vi "SPIM Controller 2016.vi"() -> ()   [LabVIEW 2016]
uses:
  controls/Microscope Settings.ctl
  controls/CameraControlTypeDef.ctl
  controls/ModeEnum.ctl
panel:
  in  "File Path Control":path
  in  "Add Settings":bool
  out "error IO":errorcluster
  out "Duration":string
  in  "Scans":dbl=1.0 min=0.0 max=10.0 step=0.05
  in  "Scan":bool
  in  "Scan Cont":bool
  in  "Multicolumn Listbox":i32(listbox)
  in  "stop":bool
  in  "Load Settings":bool
  in  "Save Settings":bool
  in  "Record":bool
  in  "Signals Debugger":bool
  in  "Stage Controller":bool
  in  "Microscope Settings":T1={"Mode"=enum."XY", "Slit"={"Scanning Mode"=12.0, "Slit Width /%"=5.0}, "Colour"=[{"Laser"=enum."561", "Filter"=4}], "Exposure/ms"=40.0, "Piezo Position /um"=0.0, "ROI"={"X"={"Start /px"=0.0, "Step /px"=1.0, "Range /px"=2048.0}, "Y"={"Start /px"=0.0, "Step /px"=1.0, "Range /px"=2048.0}, "Z "={"Start /um"=0.0, "Step/um"=1.0, "Range /um"=100.0}, "T "={"Start /s"=0.0, "Step /s"=1.0, "Range /s"=100.0}}, "Samples per millisecond"=100.0, "Relax/ms"=10.0, "Readout Direction"=2.0, "Trigger Source"=2.0, "Camera Delay /ms"=11.0, "Under Scan /ms"=5.0, "Calibration Coordinates"={"Top Left"=[-4.418670520231216, -0.1592138728323702, 10.0], "Top Right"=[-9.501965317919073, -0.1592138728323702, 10.0], "Bottom Left"=[-4.4508670520231215, 0.0, 0.0], "Bottom Right"=[-9.53757225433526, 0.0, 0.0], "Waveforms"={"Analogue Out"=[], "Digital Out"=[]}}} {"Under Scan /ms" min=0.0 max=10.0 step=0.05; "ROI"."T"."Range /s" min=0.0 max=10.0 step=0.05 format="%<%H:%M:%S>t"; "ROI"."T"."Step /s" min=0.0 max=10.0 step=0.05 format="%<%M:%S%2u>t"; "ROI"."T"."Start /s" min=0.0 max=10.0 step=0.05 format="%<%M:%S%2u>t"; "ROI"."X"."Range /px" min=0.0 max=10.0 step=0.05; "ROI"."X"."Step /px" min=0.0 max=10.0 step=0.05; "ROI"."X"."Start /px" min=0.0 max=10.0 step=0.05; "ROI"."Y"."Range /px" min=0.0 max=10.0 step=0.05; "ROI"."Y"."Step /px" min=0.0 max=10.0 step=0.05; "ROI"."Y"."Start /px" min=0.0 max=10.0 step=0.05; "ROI"."Z"."Range /um" min=0.0 max=10.0 step=0.05; "ROI"."Z"."Step/um" min=0.0001 max=10.0 step=0.05; "ROI"."Z"."Start /um" min=0.0 max=10.0 step=0.05; "Colour"."Filter" items=["Empty"=1, ""=2, ""=3, "561"=4, ""=5, "488"=6]; "Camera Delay /ms" min=0.0 max=10.0 step=0.05; "Trigger Source" items=["Internal"=1.0, "External"=2.0]; "Readout Direction" items=["Forward"=1.0, "Backward"=2.0]; "Slit"."Scanning Mode" items=["Full Frame"=1.0, "Slit Scanning"=12.0]; "Piezo Position /um" min=0.0 max=10.0 step=0.05}
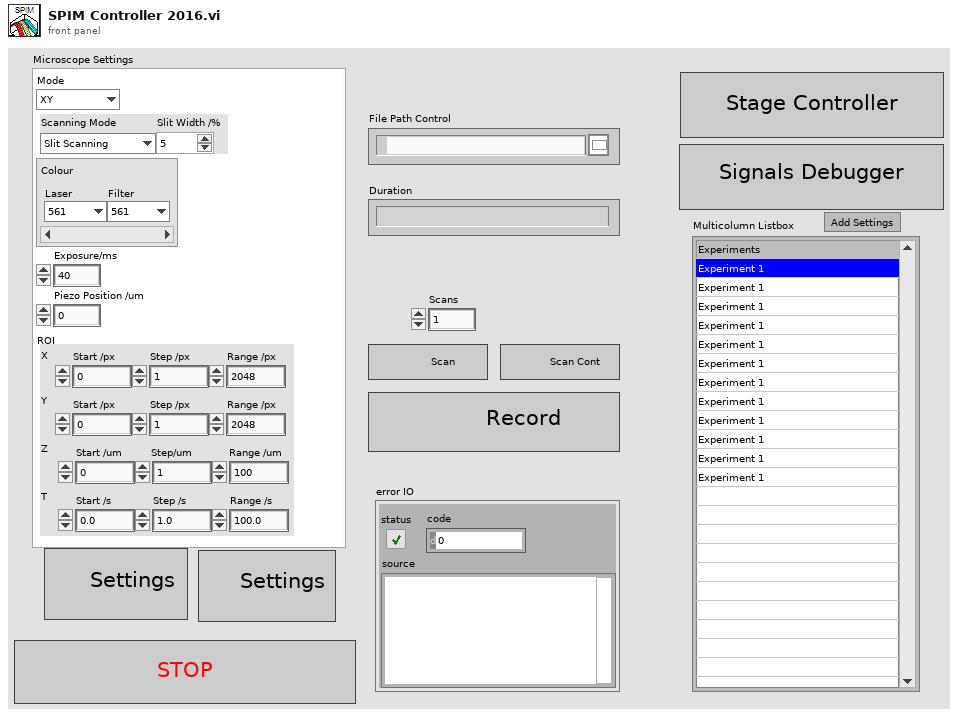
[diagram p1: front panel]
types:
  T1 = typedef "Microscope Settings.ctl" = cluster{"Mode":enum16{"Brightfield", "X", "XY", "XYZ", "XYZT", "XYZC", "Tweezers", "Virus"}, "Slit":cluster{"Scanning Mode":dbl, "Slit Width /%":dbl}, "Colour":cluster{"Laser":enum16{"Brightfield", "445", "488", "561", "647"}, "Filter":u16}[], "Exposure/ms":dbl, "Piezo Position /um":dbl, "ROI":cluster{"X":cluster{"Start /px":dbl, "Step /px":dbl, "Range /px":dbl}, "Y":cluster{"Start /px":dbl, "Step /px":dbl, "Range /px":dbl}, "Z ":cluster{"Start /um":dbl, "Step/um":dbl, "Range /um":dbl}, "T ":cluster{"Start /s":dbl, "Step /s":dbl, "Range /s":dbl}}, "Samples per millisecond":dbl, "Relax/ms":dbl, "Readout Direction":dbl, "Trigger Source":dbl, "Camera Delay /ms":dbl, "Under Scan /ms":dbl, "Calibration Coordinates":cluster{"Top Left":dbl[], "Top Right":dbl[], "Bottom Left":dbl[], "Bottom Right":dbl[], "Waveforms":cluster{"Analogue Out":waveform(dbl)[], "Digital Out":digitalwaveform[]}}}
  T2 = typedef "ModeEnum.ctl" = enum16{"Idle", "Init", "generateWaves", "runWaves", "runWavesCont", "endWavesCont", "stop"}
  T3 = typedef "CameraControlTypeDef.ctl" = enum16{"Idle", "Init", "Close", "IntervalLineInt", "Ram Record", "HardDisk Record", "Disengage Update", "Update", "ROI", "Binning", "Scan Mode", "Trigger Mode", "Readout Mode", "Readout Direction", "Preview", "ROIWindow", "Trigger Source"}
  T4 = enum32{"Invalid", "Standard", "Closed", "Hidden", "Minimized", "Maximized"}
  T5 = enum16{"open", "replace", "create", "open or create", "replace or create", "replace or create with confirmation"}
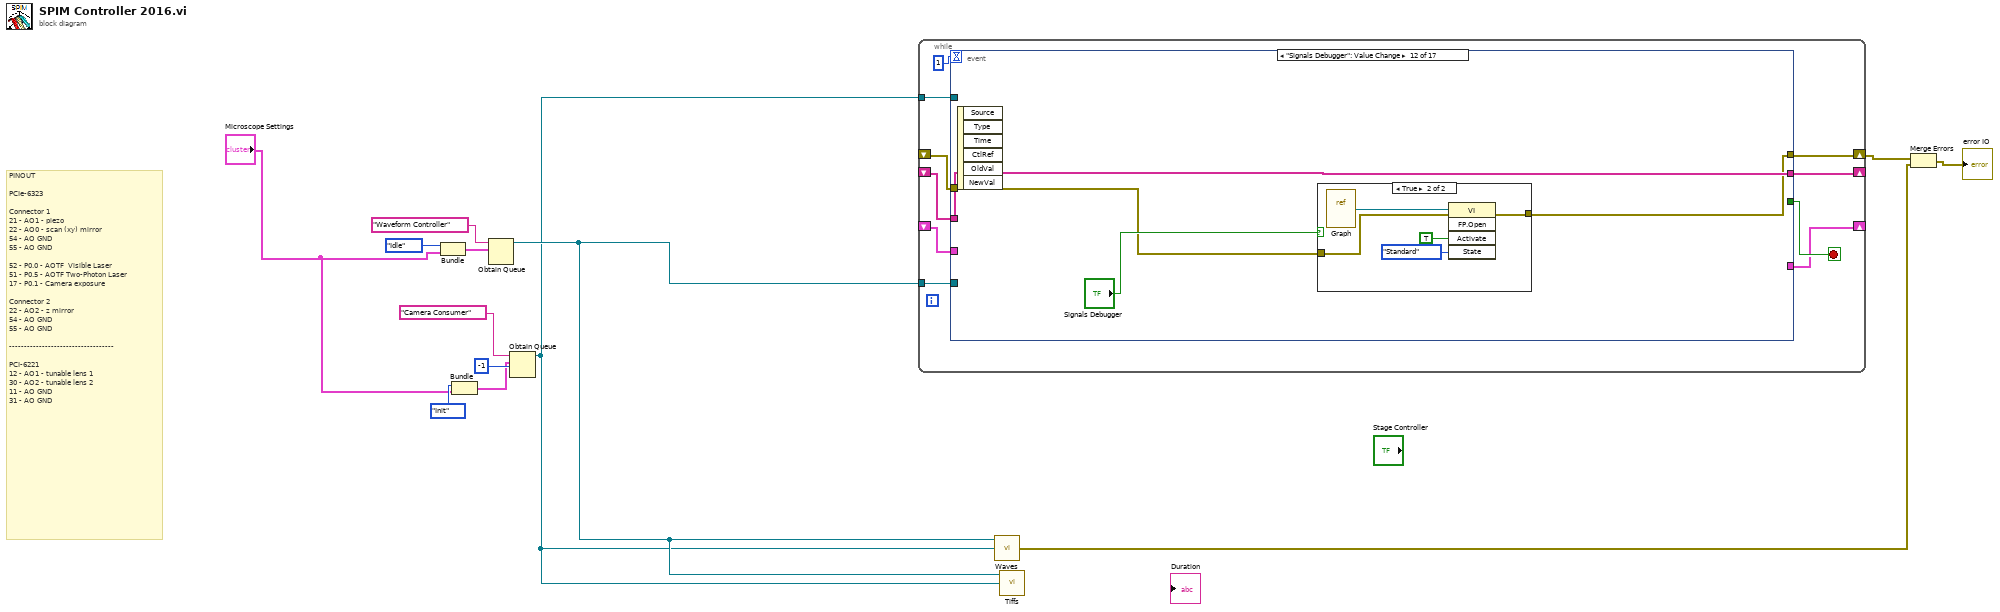
[diagram p0: block diagram]
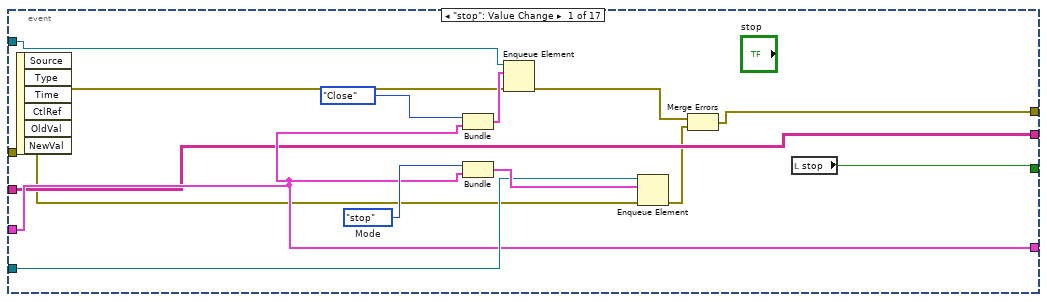
[diagram p2: hidden frame]
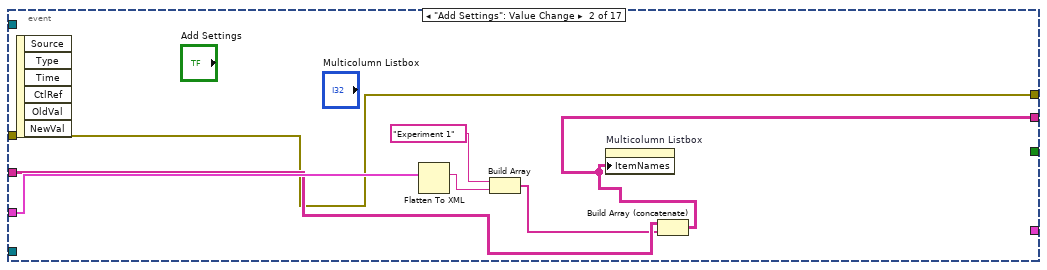
[diagram p3: hidden frame]
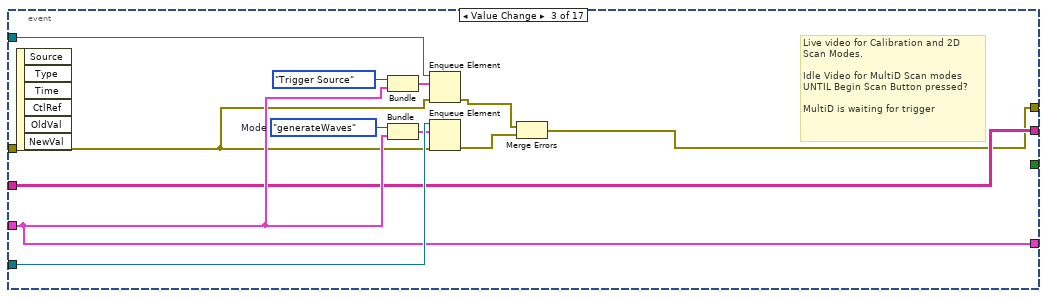
[diagram p4: hidden frame]
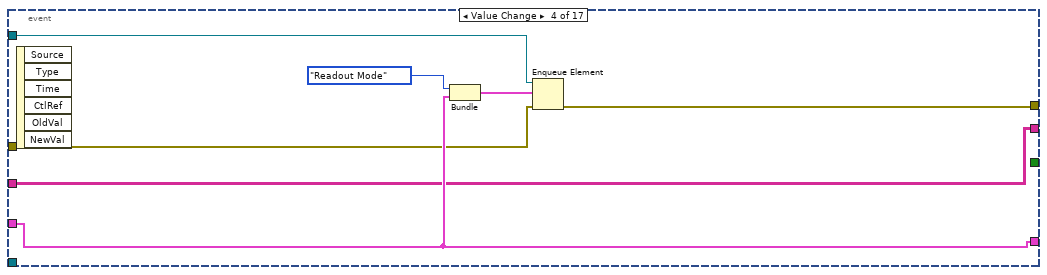
[diagram p5: hidden frame]
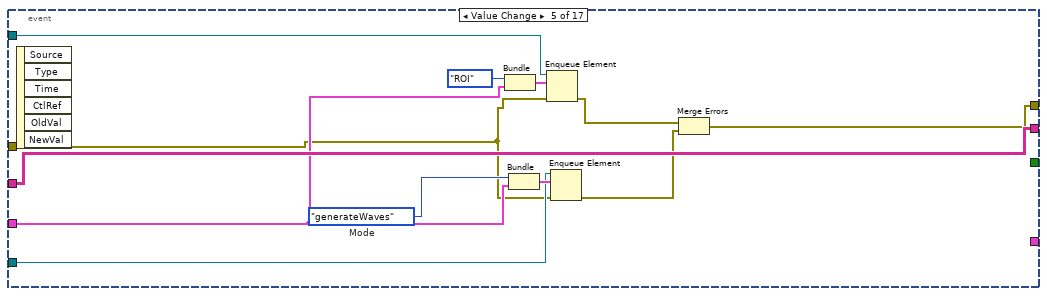
[diagram p6: hidden frame]
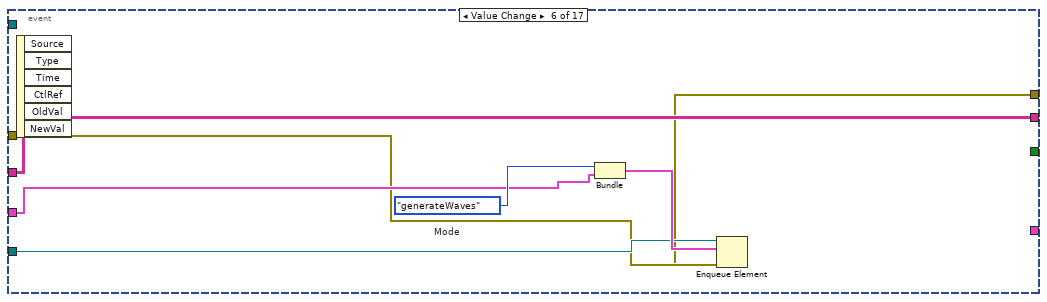
[diagram p7: hidden frame]
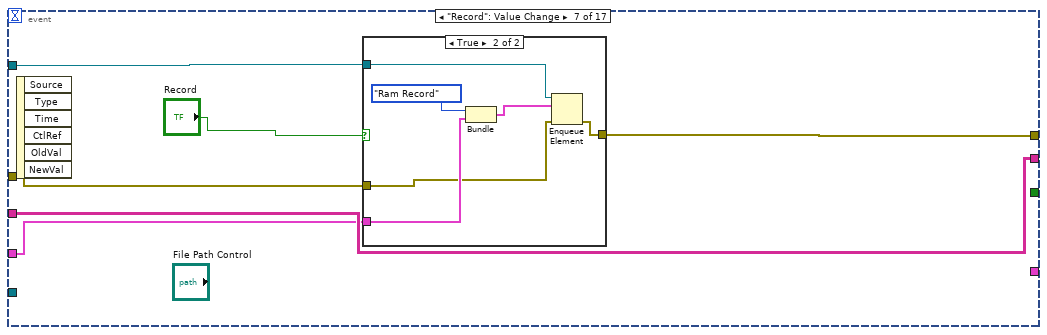
[diagram p8: hidden frame]
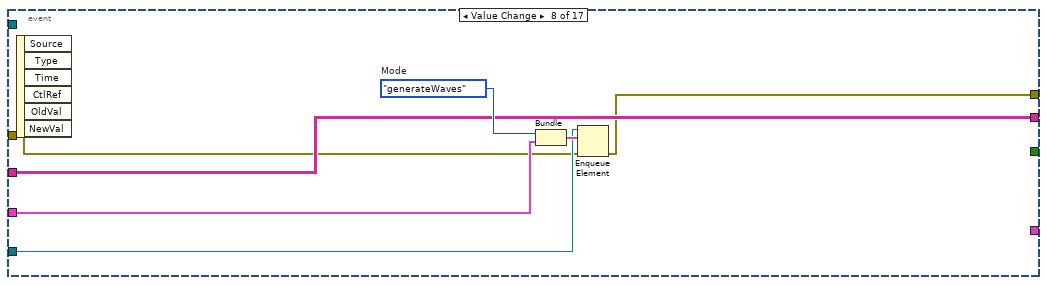
[diagram p10: hidden frame]
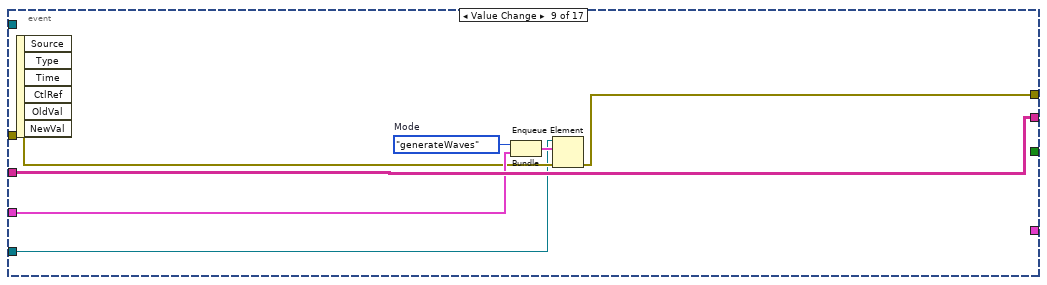
[diagram p11: hidden frame]
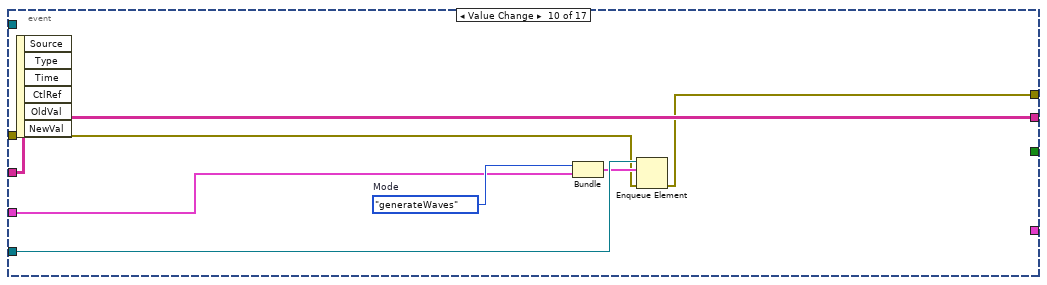
[diagram p12: hidden frame]
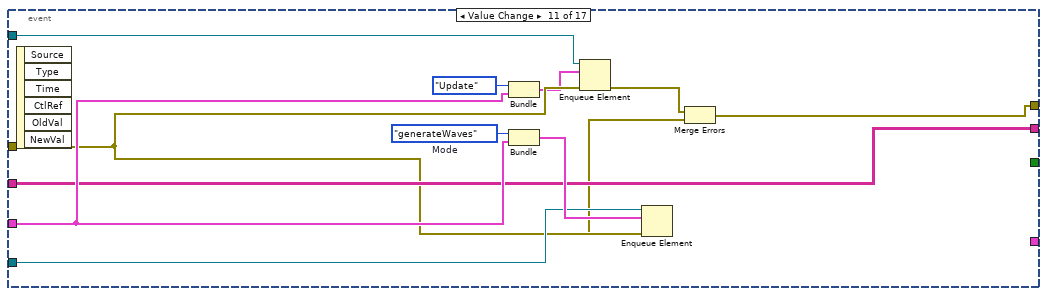
[diagram p13: hidden frame]
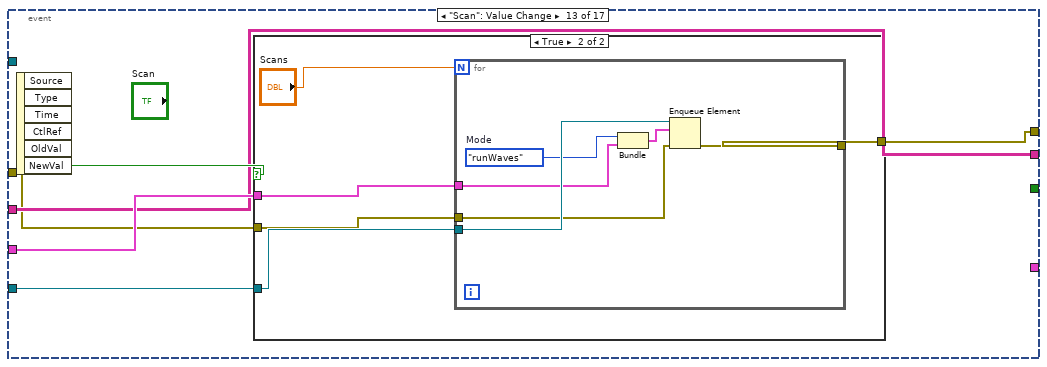
[diagram p15: hidden frame]
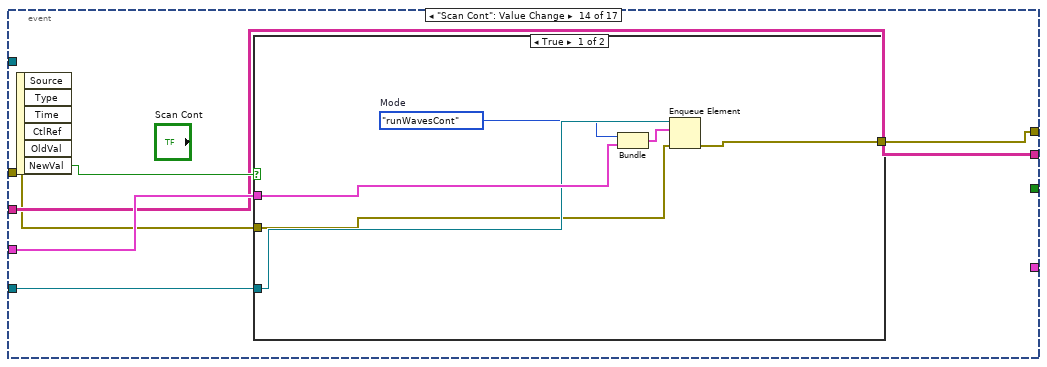
[diagram p17: hidden frame]
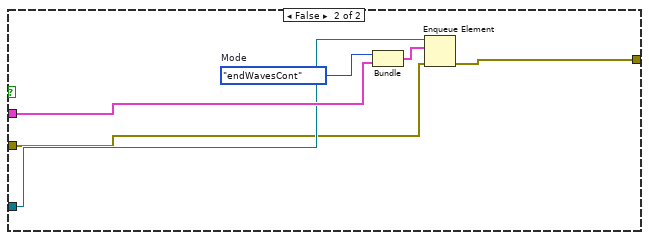
[diagram p18: hidden frame]
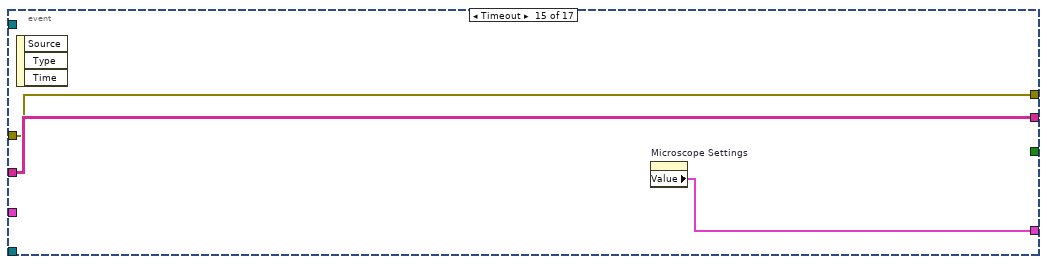
[diagram p19: hidden frame]
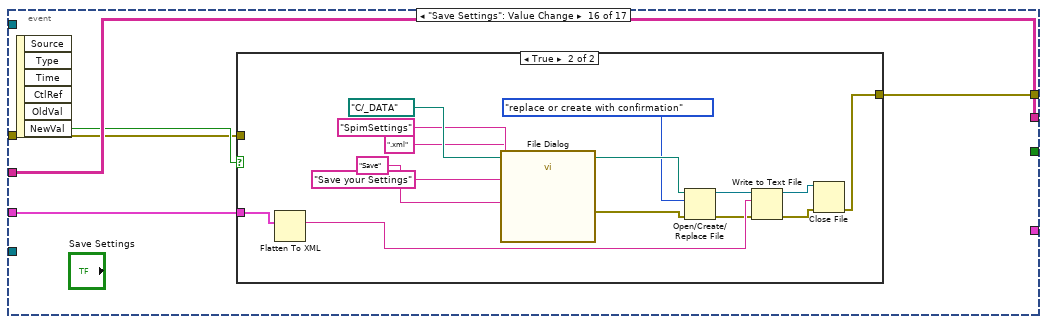
[diagram p20: hidden frame]
diagram:
  # "PINOUT\n\nPCIe-6323\n\nConnector 1\n21 - AO1 - piezo\n22 - AO0 - scan (xy) mirror\n54 - AO GND\n55 - AO GND\n\n52 - P0.0 - AOTF  Visible Laser\n51 - P0.5 - AOTF Two-Photon Laser\n17 - P0.1 - Camera exposure\n\nConnector 2\n22 - AO2 - z mirror\n54 - AO GND\n55 - AO GND\n\n-----------------------------------\n\nPCI-6221\n12 - AO1 - tunable lens 1\n30 - AO2 - tunable lens 2\n11 - AO GND\n31 - AO GND"
  n1 = Bundle("Mode"=ModeEnum."Idle", "Microscope Settings"="Microscope Settings") -> (w8:cluster{"Mode":T2, "Microscope Settings":T1})  [unwired: 1 in]
  n2 = Bundle("Enum"=CameraControlTypeDef."Init", "Microscope Settings"="Microscope Settings") -> (w10:cluster{"Enum":T3, "Microscope Settings":T1})  [unwired: 1 in]
  n3 = Obtain Queue(name (unnamed)="Waveform Controller", element data type=w8) -> (queue out=w6:refnum<queue>)  [unwired: 3 in, 2 out]
  n4 = Obtain Queue(max queue size (-1, unlimited)=-1, name (unnamed)="Camera Consumer", element data type=w10) -> (queue out=w5:refnum<queue>)  [unwired: 2 in, 2 out]
  n5 = while {
    tunnel: w5 -> [w22]
    shift-right: [w21] -> _
    shift-left: _ -> [w20]
    tunnel: w6 -> [w18]
    shift-right: [w17] -> _
    shift-left: _ -> [w16]
    shift-right: [w15] -> w3
    shift-left: _ -> [w14]
    stop <- w23 stop-if-true
    n6 = event shown="[11] \"Signals Debugger\": Value Change" {
      selector: _ -> [_ _ _ _ _ _ _ _ _ _ _ _ _ _ _ _ _]
      dyn-events: _ -> [_ _ _ _ _ _ _ _ _ _ _ _ _ _ _ _ _]
      timeout: 1 -> [_ _ _ _ _ _ _ _ _ _ _ _ _ _ _ _ _]
      tunnel: [w36 _ _ _ _ _ _ _ _ _ _ _ _ _ _ _ _] -> w23
      tunnel: w22 -> [w24 _ w44 w56 w63 _ w86 _ _ _ w116 _ _ _ _ _ _]
      tunnel: [w30 _ w50 w61 _ _ _ _ _ _ _ _ _ _ w176 _ w199] -> w21
      tunnel: w20 -> [w30 w43 w50 w61 w69 w77 w85 w99 w106 w112 w124 _ w143 w161 _ w180 w200]
      tunnel: w18 -> [w31 _ w55 _ w70 w78 _ w98 w102 w113 w123 _ w142 w160 _ _ _]
      tunnel: [w29 w38 w49 w59 w72 w81 w87 w97 w108 w115 w122 w131 w140 w158 w175 w181 w201] -> w17
      tunnel: w16 -> [w29 w40 w49 w59 w72 w81 w87 w97 w108 w115 w122 w131 w140 w158 w175 w181 w201]
      tunnel: [w25 w37 w45 w57 w64 w75 w83 w95 w104 w110 w118 w129 w139 w157 w174 w179 _] -> w15
      tunnel: w14 -> [w28 w37 w48 w58 w67 w76 w84 w96 w105 w109 w121 w128 w138 w156 w174 w177 _]
      event "stop": Value Change {
        w34 = ModeEnum."stop"  # Mode
        n7 = event-data() -> ()  [unwired: 1 in, 6 out]
        n8 = Bundle("Enum"=CameraControlTypeDef."Close", "Value"=w30) -> (w32:cluster{"Enum":T3, "Value":T1})  [unwired: 1 in]
        n9 = Bundle("Mode"=w34, "Value"=w30) -> (w33:cluster{"Mode":T2, "Value":T1})  [unwired: 1 in]
        n10 = Enqueue Element(queue=w24, element=w32, error in (no error)=w28) -> (error out=w26:errorcluster)  [unwired: 1 in, 2 out]
        n11 = Enqueue Element(queue=w31, element=w33, error in (no error)=w28) -> (error out=w27:errorcluster)  [unwired: 1 in, 2 out]
        n12 = Merge Errors(w26, w27) -> (w25:errorcluster)
        n13 = local read "stop"() -> (w36:bool)
      }
      event "Add Settings": Value Change {
        n14 = event-data() -> ()  [unwired: 1 in, 6 out]
        n15 = Flatten To XML(anything=w43) -> (xml string=w42:string)
        n16 = Build Array("Experiment 1" ("element"), w42) -> (w39:string[])
        n17 = Build Array (concatenate)(w40, w39) -> (w38:string[][])
        n18 = property on="Multicolumn Listbox" class="MCListbox (strict)"("ItemNames"=w38) -> ()  [unwired: 2 in, 2 out]
      }
      event Value Change {
        w53 = ModeEnum."generateWaves"  # Mode
        # "Live video for Calibration and 2D\nScan Modes.\n\nIdle Video for MultiD Scan modes\nUNTIL Begin Scan Button pressed?\n\nMultiD is waiting for trigger"
        n19 = event-data() -> ()  [unwired: 1 in, 6 out]
        n20 = Bundle("Enum"=CameraControlTypeDef."Trigger Source", "Value"=w50) -> (w51:cluster{"Enum":T3, "Value":T1})  [unwired: 1 in]
        n21 = Bundle("Mode"=w53, "Value"=w50) -> (w52:cluster{"Mode":T2, "Value":T1})  [unwired: 1 in]
        n22 = Enqueue Element(queue=w44, element=w51, error in (no error)=w48) -> (error out=w46:errorcluster)  [unwired: 1 in, 2 out]
        n23 = Enqueue Element(queue=w55, element=w52, error in (no error)=w48) -> (error out=w47:errorcluster)  [unwired: 1 in, 2 out]
        n24 = Merge Errors(w46, w47) -> (w45:errorcluster)
      }
      event Value Change {
        n25 = event-data() -> ()  [unwired: 1 in, 6 out]
        n26 = Bundle("Enum"=CameraControlTypeDef."Readout Mode", "Value"=w61) -> (w60:cluster{"Enum":T3, "Value":T1})  [unwired: 1 in]
        n27 = Enqueue Element(queue=w56, element=w60, error in (no error)=w58) -> (error out=w57:errorcluster)  [unwired: 1 in, 2 out]
      }
      event Value Change {
        w68 = ModeEnum."generateWaves"  # Mode
        n28 = event-data() -> ()  [unwired: 1 in, 6 out]
        n29 = Bundle("Enum"=CameraControlTypeDef."ROI", "Value"=w69) -> (w73:cluster{"Enum":T3, "Value":T1})  [unwired: 1 in]
        n30 = Bundle("Mode"=w68, "Value"=w69) -> (w71:cluster{"Mode":T2, "Value":T1})  [unwired: 1 in]
        n31 = Enqueue Element(queue=w63, element=w73, error in (no error)=w67) -> (error out=w65:errorcluster)  [unwired: 1 in, 2 out]
        n32 = Enqueue Element(queue=w70, element=w71, error in (no error)=w67) -> (error out=w66:errorcluster)  [unwired: 1 in, 2 out]
        n33 = Merge Errors(w65, w66) -> (w64:errorcluster)
      }
      event Value Change {
        w79 = ModeEnum."generateWaves"  # Mode
        n34 = event-data() -> ()  [unwired: 1 in, 6 out]
        n35 = Bundle("Mode"=w79, "Value"=w77) -> (w80:cluster{"Mode":T2, "Value":T1})  [unwired: 1 in]
        n36 = Enqueue Element(queue=w78, element=w80, error in (no error)=w76) -> (error out=w75:errorcluster)  [unwired: 1 in, 2 out]
      }
      event "Record": Value Change {
        n37 = event-data() -> ()  [unwired: 1 in, 6 out]
        n38 = case shown="True" "Record" {
          tunnel: w86 -> [_ w89]
          tunnel: w85 -> [_ w93]
          tunnel: w84 -> [w88 w91]
          tunnel: [w88 w90] -> w83
          frame False {
          }
          frame True {
            n39 = Bundle("Enum"=CameraControlTypeDef."Ram Record", "Value"=w93) -> (w92:cluster{"Enum":T3, "Value":T1})  [unwired: 1 in]
            n40 = Enqueue Element(queue=w89, element=w92, error in (no error)=w91) -> (error out=w90:errorcluster)  [unwired: 1 in, 2 out]
          }
        }
      }
      event Value Change {
        w101 = ModeEnum."generateWaves"  # Mode
        n41 = event-data() -> ()  [unwired: 1 in, 6 out]
        n42 = Bundle("Mode"=w101, "Value"=w99) -> (w100:cluster{"Mode":T2, "Value":T1})  [unwired: 1 in]
        n43 = Enqueue Element(queue=w98, element=w100, error in (no error)=w96) -> (error out=w95:errorcluster)  [unwired: 1 in, 2 out]
      }
      event Value Change {
        w107 = ModeEnum."generateWaves"  # Mode
        n44 = event-data() -> ()  [unwired: 1 in, 6 out]
        n45 = Bundle("Mode"=w107, "Value"=w106) -> (w103:cluster{"Mode":T2, "Value":T1})  [unwired: 1 in]
        n46 = Enqueue Element(queue=w102, element=w103, error in (no error)=w105) -> (error out=w104:errorcluster)  [unwired: 1 in, 2 out]
      }
      event Value Change {
        w114 = ModeEnum."generateWaves"  # Mode
        n47 = event-data() -> ()  [unwired: 1 in, 6 out]
        n48 = Bundle("Mode"=w114, "Value"=w112) -> (w111:cluster{"Mode":T2, "Value":T1})  [unwired: 1 in]
        n49 = Enqueue Element(queue=w113, element=w111, error in (no error)=w109) -> (error out=w110:errorcluster)  [unwired: 1 in, 2 out]
      }
      event Value Change {
        w126 = ModeEnum."generateWaves"  # Mode
        n50 = event-data() -> ()  [unwired: 1 in, 6 out]
        n51 = Bundle("Enum"=CameraControlTypeDef."Update", "Value"=w124) -> (w117:cluster{"Enum":T3, "Value":T1})  [unwired: 1 in]
        n52 = Bundle("Mode"=w126, "Value"=w124) -> (w125:cluster{"Mode":T2, "Value":T1})  [unwired: 1 in]
        n53 = Enqueue Element(queue=w116, element=w117, error in (no error)=w121) -> (error out=w120:errorcluster)  [unwired: 1 in, 2 out]
        n54 = Enqueue Element(queue=w123, element=w125, error in (no error)=w121) -> (error out=w119:errorcluster)  [unwired: 1 in, 2 out]
        n55 = Merge Errors(w120, w119) -> (w118:errorcluster)
      }
      event "Signals Debugger": Value Change {
        n56 = event-data() -> ()  [unwired: 1 in, 6 out]
        n57 = case shown="True" "Signals Debugger" {
          tunnel: [w132 w134] -> w129
          tunnel: w128 -> [w132 w133]
          frame False {
          }
          frame True {
            n58 = vi-ref "Graph.vi"() -> (w135:refnum<vi>)
            n59 = invoke class="VI" method="FP.Open"(reference=w135, error in=w133, "Activate"=TRUE ("Front Panel Window:Open"), "State"=T4."Standard") -> (error out=w134:errorcluster)  [unwired: 1 in, 4 out]
          }
        }
      }
      event "Scan": Value Change {
        n60 = event-data() -> ("NewVal"=w141:bool)  [unwired: 1 in, 5 out]
        n61 = case shown="True" w141 {
          tunnel: w143 -> [_ w149]
          tunnel: w142 -> [_ w148]
          tunnel: [w144 w147] -> w139
          tunnel: w138 -> [w144 w146]
          frame False {
          }
          frame True {
            n62 = for {
              N: "Scans" -> [_]
              tunnel: w149 -> [w152]
              tunnel: w148 -> [w155]
              tunnel: [w151] -> w147
              tunnel: w146 -> [w150]
              w154 = ModeEnum."runWaves"  # Mode
              n63 = Bundle("Mode"=w154, "Value"=w152) -> (w153:cluster{"Mode":T2, "Value":T1})  [unwired: 1 in]
              n64 = Enqueue Element(queue=w155, element=w153, error in (no error)=w150) -> (error out=w151:errorcluster)  [unwired: 1 in, 2 out]
            }
          }
        }
      }
      event "Scan Cont": Value Change {
        n65 = event-data() -> ("NewVal"=w159:bool)  [unwired: 1 in, 5 out]
        n66 = case shown="True" w159 {
          tunnel: w161 -> [w167 w173]
          tunnel: w160 -> [w166 w172]
          tunnel: [w165 w171] -> w157
          tunnel: w156 -> [w164 w170]
          frame True {
            w163 = ModeEnum."runWavesCont"  # Mode
            n67 = Bundle("Mode"=w163, "Value"=w167) -> (w162:cluster{"Mode":T2, "Value":T1})  [unwired: 1 in]
            n68 = Enqueue Element(queue=w166, element=w162, error in (no error)=w164) -> (error out=w165:errorcluster)  [unwired: 1 in, 2 out]
          }
          frame False {
            w169 = ModeEnum."endWavesCont"  # Mode
            n69 = Bundle("Mode"=w169, "Value"=w173) -> (w168:cluster{"Mode":T2, "Value":T1})  [unwired: 1 in]
            n70 = Enqueue Element(queue=w172, element=w168, error in (no error)=w170) -> (error out=w171:errorcluster)  [unwired: 1 in, 2 out]
          }
        }
      }
      event Timeout {
        n71 = event-data() -> ()  [unwired: 1 in, 3 out]
        n72 = property on="Microscope Settings" class="Clust (strict)"() -> ("Value"=w176:T1)  [unwired: 2 in, 2 out]
      }
      event "Save Settings": Value Change {
        n73 = event-data() -> ("NewVal"=w178:bool)  [unwired: 1 in, 5 out]
        n74 = case shown="True" w178 {
          tunnel: w180 -> [_ w197]
          tunnel: [w182 w185] -> w179
          tunnel: w177 -> [w182 _]
          frame False {
          }
          frame True {
            n75 = Flatten To XML(anything=w197) -> (xml string=w190:string)
            n76 = call "File Dialog"("start path"=path "C:/_DATA", "prompt"="Save your Settings", "button label"="Save", "default name"="SpimSettings", "pattern (all files)"=".xml") -> ("selected path"=w191:path, "error out"=w184:errorcluster)  [unwired: 7 in, 2 out]
            n77 = Open/Create/Replace File(file path (use dialog)=w191, error in=w184, operation (0:open)=T5."replace or create with confirmation") -> (refnum out=w189:refnum<file>, error out=w186:errorcluster)  [unwired: 3 in, 1 out]
            n78 = Write to Text File(file (use dialog)=w189, text=w190, error in=w186) -> (refnum out=w188:refnum<file>, error out=w187:errorcluster)  [unwired: 1 in, 1 out]
            n79 = Close File(refnum=w188, error in=w187) -> (error out=w185:errorcluster)  [unwired: 1 out]
          }
        }
      }
      event "Load Settings": Value Change {
        n80 = event-data() -> ("NewVal"=w198:bool)  [unwired: 1 in, 5 out]
        n81 = case shown="True" w198 {
          tunnel: w200 -> [w202 w205]
          tunnel: [w202 w204] -> w199
          frame False {
          }
          frame True {
            (unwired) "Load your Settings" ("prompt")
            n82 = call "File Open"("start path"=path "C:/_DATA", "button label"="Load", "default name"="SpimSettings", "pattern (all files)"="*.xml") -> ("selected path"=w206:path, "cancelled"=w203:bool)  [unwired: 8 in, 2 out]
            n83 = case shown="False" w203 {
              tunnel: w206 -> [_ w216]
              tunnel: w205 -> [w211 w214]
              tunnel: [w211 w212] -> w204
              frame True {
              }
              frame False {
                n84 = Read from Text File(file (use dialog)=w216) -> (text=w215:string, error out=w213:errorcluster)  [unwired: 3 in, 2 out]
                n85 = Unflatten From XML(xml string=w215, type=w214, error in (no error)=w213) -> (value=w212:T1)  [unwired: 1 out]
                n86 = property on="Microscope Settings" class="Clust (strict)"("Val(Sgnl)"=w212) -> ()  [unwired: 2 in, 2 out]
              }
            }
          }
        }
      }
    }
  }
  n87 = call "Waves.vi"("Camera Queue"=w5, "Wave Queue"=w6) -> ("error IO"=w2:errorcluster)  [unwired: 1 in]
  n88 = call "Tiffs.vi"("Camera Queue"=w5, "Wave Queue"=w6) -> ()  [unwired: 1 in, 1 out]
  n89 = Merge Errors(w3, w2) -> (→"error IO":errorcluster)
